vi "initHelpButtonVisibility.vi"(9 "error in":errorcluster, 11 "Help":refnum<vi>) -> (1 "error out":errorcluster)   [LabVIEW 2017]
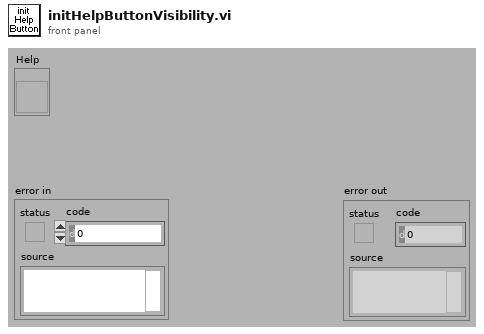
[diagram p1: front panel]
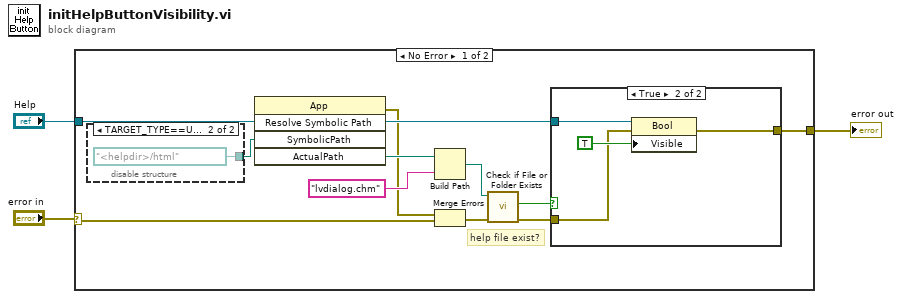
[diagram p0: block diagram]
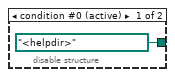
[diagram p2: hidden frame]
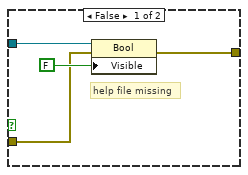
[diagram p3: hidden frame]
diagram:
  n1 = case shown="No Error" "error in" {
    selector: "error in" -> [w5 w25]
    tunnel: [w10 w25] -> w2
    tunnel: "Help" -> [w9 _]
    frame No Error {
      # "help file exist?"
      n2 = disable-structure shown="TARGET_TYPE==Unix||TARGET_TYPE==Mac" {
        disable-tunnel: [path "<helpdir>" ("base path") path "<helpdir>/html" ("base path")] -> w8
        frame condition #0 (active) {
        }
        frame condition #1 {
        }
      }
      n3 = invoke class="App" method="Resolve Symbolic Path"("SymbolicPath"=w8) -> (error out=w6:errorcluster, "ActualPath"=w7:path)  [unwired: 4 in, 3 out]
      n4 = Build Path(base path=w7, name or relative path="lvdialog.chm" ("CHM or HLP filename (lvdialog.chm)")) -> (appended path=w13:path)
      n5 = Merge Errors(w6, w5) -> (w4:errorcluster)
      n6 = call <vilib>:"Check if File or Folder Exists.vi"("error in (no error)"=w4, "path"=w13) -> ("error out"=w11:errorcluster, "file or folder exists?"=w12:bool)  [unwired: 8 out]
      n7 = case shown="True" w12 {
        tunnel: [w17 w21] -> w10
        tunnel: w11 -> [w18 w22]
        tunnel: w9 -> [w19 w24]
        frame False {
          # "help file missing"
          n8 = property class="Bool"(reference=w19, error in=w18, "Visible"=FALSE) -> (error out=w17:errorcluster)  [unwired: 1 out]
        }
        frame True {
          n9 = property class="Bool"(reference=w24, error in=w22, "Visible"=TRUE) -> (error out=w21:errorcluster)  [unwired: 1 out]
        }
      }
    }
    frame Error {
    }
  }
  "error out" <- w2
